vi "Array differences Int.vi"(8 "Array 2":i32[](array[numeric]), 11 "Array 1":i32[](array[numeric])) -> (0 "Komplement Array 2":i32[](array[numeric]), 3 "Komplement Array 1":i32[](array[numeric]))   [LabVIEW 2017, in "util.lvlib"]
uses:
  util.lvlib
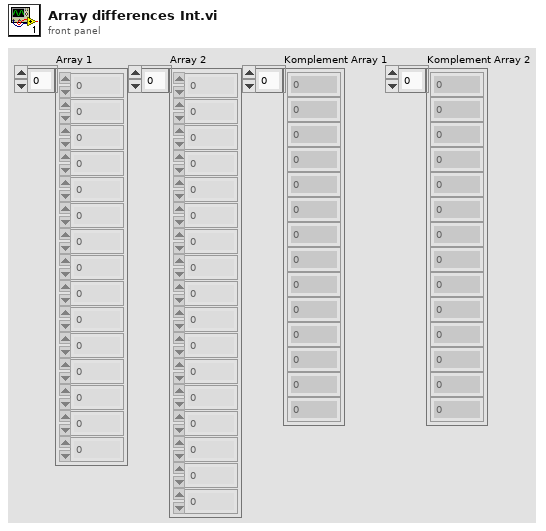
[diagram p1: front panel]
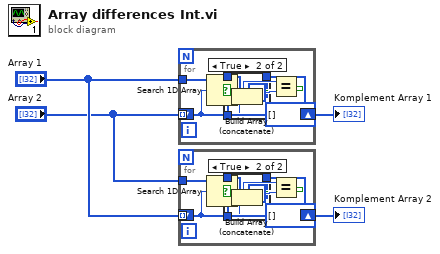
[diagram p0: block diagram]
diagram:
  n1 = for {
    tunnel: "Array 2" -> [w10] mode=indexing
    tunnel: "Array 1" -> [w13]
    shift-right: [w7] -> w6
    shift-left: i32[] [] ("Array") -> [w8]
    n2 = Search 1D Array(1D array=w13, element=w10) -> (index of element=w12:i32)  [unwired: 1 in]
    n3 = Equal?(x=w12, y=-1) -> (x = y?=w9:bool)
    n4 = case shown="True" w9 {
      tunnel: w8 -> [w14 w16]
      tunnel: w10 -> [_ w15]
      tunnel: [w14 w17] -> w7
      frame False {
      }
      frame True {
        n5 = Build Array (concatenate)(w16, w15) -> (w17:i32[])
      }
    }
  }
  "Komplement Array 1" <- w6
  n6 = for {
    tunnel: "Array 1" -> [w21] mode=indexing
    tunnel: "Array 2" -> [w24]
    shift-right: [w18] -> w5
    shift-left: i32[] [] ("Array") -> [w19]
    n7 = Search 1D Array(1D array=w24, element=w21) -> (index of element=w23:i32)  [unwired: 1 in]
    n8 = Equal?(x=w23, y=-1) -> (x = y?=w20:bool)
    n9 = case shown="True" w20 {
      tunnel: w19 -> [w25 w27]
      tunnel: w21 -> [_ w26]
      tunnel: [w25 w28] -> w18
      frame False {
      }
      frame True {
        n10 = Build Array (concatenate)(w27, w26) -> (w28:i32[])
      }
    }
  }
  "Komplement Array 2" <- w5
